vi "Assert One Of.vi"(7 "Label":string="Assert One Of", 8 "error in (no error)":errorcluster, 10 "Actual":variant, 11 "Options":variant[](array[variant])) -> (0 "error out":errorcluster)   [LabVIEW 2017, in "Assert Extensions.lvclass"]
uses:
  Assert Extensions.lvclass
  6c9e5f8f-5649-40c7-97ba-bf585a19c4df.vi
  3b3e265a-5e95-42c1-a134-ca2746af6ef6.vi
  <vilib>/addons/_JKI Toolkits/Caraya/classes/Properties.Assert/Properties.Assert.lvclass
  C:/Program Files/National Instruments/LabVIEW 2017/vi.lib/addons/_JKI Toolkits/Caraya/classes/Properties/Properties.lvclass
  <vilib>/JDP Science/JSONtext/Variant to JSON Text.vi
  <vilib>/JDP Science/JSONtext/LVClass Serializer/JSONtext LVClass Serializer.lvclass
  <vilib>/addons/_JKI Toolkits/Caraya/classes/Assert/Assert.lvclass
  <vilib>/addons/_JKI Toolkits/Caraya/classes/Properties/Properties.lvclass
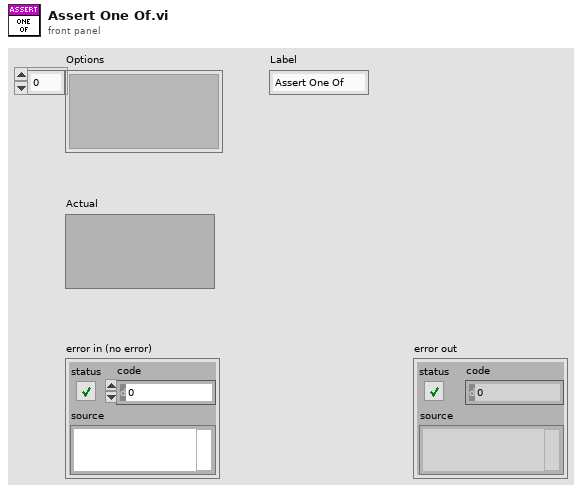
[diagram p1: front panel]
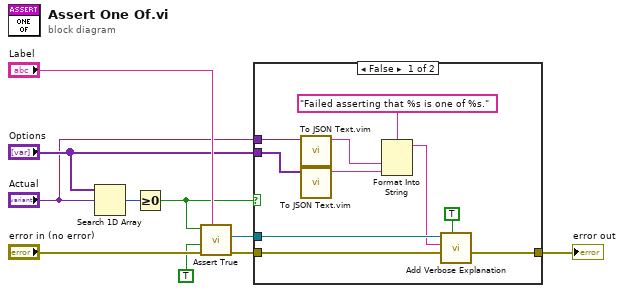
[diagram p0: block diagram]
diagram:
  n1 = Search 1D Array(1D array="Options", element="Actual") -> (index of element=w9:i32)  [unwired: 1 in]
  n2 = Greater Or Equal To 0?(x=w9) -> (x >= 0?=w4:bool)
  n3 = call <vilib>:"Assert True.vi"("Label"="Label", "error in (no error)"="error in (no error)", "Register with caller test (F)"=TRUE, "True?"=w4) -> ("error out"=w6:errorcluster, "Properties"=w3:refnum<class "Properties.Assert.lvclass">)  [unwired: 6 in]
  n4 = case shown="False" w4 {
    tunnel: w6 -> [w19 w21]
    tunnel: [w18 w21] -> w5
    tunnel: w3 -> [w17 _]
    tunnel: "Options" -> [w12 _]
    tunnel: "Actual" -> [w14 _]
    frame False {
      n5 = call "To JSON Text.vim"("Anything"=w14) -> ("<JSON>"=w13:string)  [unwired: 9 in, 1 out]
      n6 = call "To JSON Text.vim"("Anything"=w12) -> ("<JSON>"=w11:string)  [unwired: 9 in, 1 out]
      n7 = Format Into String(format string="Failed asserting that %s is one of %s.", w13, w11) -> (resulting string=w15:string)  [unwired: 2 in, 1 out]
      n8 = call <vilib>:"Add Verbose Explanation.vi"("overwrite?"=TRUE, "error in (no error)"=w19, "Verbose Explanation"=w15, "Properties"=w17) -> ("error out"=w18:errorcluster)  [unwired: 6 in, 1 out]
    }
    frame True {
    }
  }
  "error out" <- w5
